vi "Create ArrayVarying.vi"(8 "error in (no error)":errorcluster, 11 "Scanner.lvclass":refnum<class "Scanner.lvclass">) -> (0 "error out":errorcluster, 2 "# Points":u32, 3 "Scanner.lvclass out":refnum<class "Scanner.lvclass">)   [LabVIEW 2009, in "Scanner.lvclass"]
doc: "Generate an internal array of independent variables from the Range. You do not need to use this array if it makes no sense for your subclass; it is merely provided for convenience."
uses:
  Scanner.lvclass
  Scanner.lvclass/Scanner.ctl
panel:
  out "Ind Vars":dbl[](array[numeric])
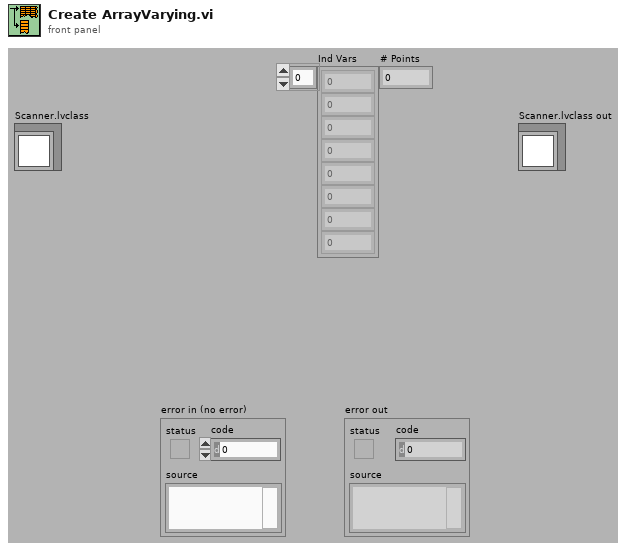
[diagram p1: front panel]
types:
  T1 = typedef "Scanner.lvclass/Range.ctl" = cluster{"xi":dbl, "xf":dbl, "dx":dbl, "Return to start?":bool}
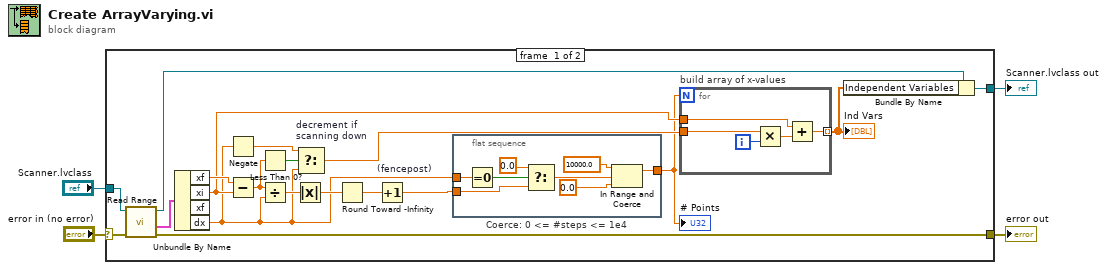
[diagram p0: block diagram]
diagram:
  n1 = case shown="No Error" "error in (no error)" {
    selector: "error in (no error)" -> [w19 w37]
    tunnel: [w23 w38] -> w4
    tunnel: "Scanner.lvclass" -> [w20 w38]
    tunnel: [w16 w37] -> w1
    frame #0 {
      n2 = call-dynamic "Read Range.vi"("error in (no error)"=w19, "Scanner.lvclass in"=w20) -> ("error out"=w16:errorcluster, "Range"=w12:T1, "Scanner.lvclass out"=w17:refnum<class "Scanner.lvclass">)  [unwired: 7 out]
      n3 = Unbundle By Name(w12) -> ("xf"=w10:dbl, "xi"=w8:dbl, "dx"=w5:dbl)  [unwired: 1 out]
      n4 = Negate(x=w5) -> (-x=w11:dbl)
      n5 = Subtract(x=w10, y=w8) -> (x-y=w9:dbl)
      n6 = Less Than 0?(x=w9) -> (x < 0?=w21:bool)
      n7 = Divide(x=w9, y=w5) -> (x/y=w14:dbl)
      n8 = Absolute Value(x=w14) -> (abs(x)=w15:dbl)
      n9 = Select "decrement if\nscanning down"(t=w11, s=w21, f=w5) -> (s? t:f=w22:dbl)
      n10 = Round Toward -Infinity(1:w15) -> (0:w13:dbl)
      n11 = Increment "(fencepost)"(x=w13) -> (x+1=w6:dbl)
      n12 = flat-sequence "Coerce: 0 <= #steps <= 1e4" {
        tunnel: [w29] -> w7
        tunnel: w6 -> [w28]
        tunnel: w5 -> [w24]
        frame #0 {
          n13 = Equal To 0?(x=w24) -> (x = 0?=w26:bool)
          n14 = Select(t=0.0, s=w26, f=w28) -> (s? t:f=w27:dbl)
          n15 = In Range and Coerce(upper limit=10000.0, x=w27, lower limit=0.0 ("upper limit")) -> (coerced(x)=w29:dbl)  [unwired: 1 out]
        }
      }
      n16 = for "build array of x-values" {
        N: w7 -> [_]
        tunnel: w8 -> [w36]
        tunnel: w22 -> [w34]
        tunnel: [w32] -> w18 mode=indexing
        i -> [w35]
        n17 = Multiply(x=w34, y=w35) -> (x*y=w33:dbl)
        n18 = Add(x=w36, y=w33) -> (x+y=w32:dbl)
      }
      "Ind Vars" <- w18
      n19 = Bundle By Name(cluster=w17, "Independent Variables"=w18) -> (w23:refnum<class "Scanner.lvclass">)
      "# Points" <- w7
    }
    frame #1 {
    }
  }
  "Scanner.lvclass out" <- w4
  "error out" <- w1
